vi "Getter.vi"(8 "Error In":errorcluster, 11 "Waypoint In":refnum<class "Waypoint.lvclass">) -> (0 "Error Out":errorcluster, 1 "Coords":T1 {"North" format="%#_10f"; "East" format="%#_8f"}, 2 "Tolerance (meters?)":dbl, 3 "Waypoint Out":refnum<class "Waypoint.lvclass">, 5 "Done?":bool)   [LabVIEW 2013, in "Waypoint.lvclass"]
doc: "A getter vi for waypoint class\n\nMac-I Crowell\nJanuray 2014"
uses:
  Waypoint.lvclass
  Data/TypeDefs/UTM Location.ctl
  Waypoint.lvclass/Waypoint.ctl
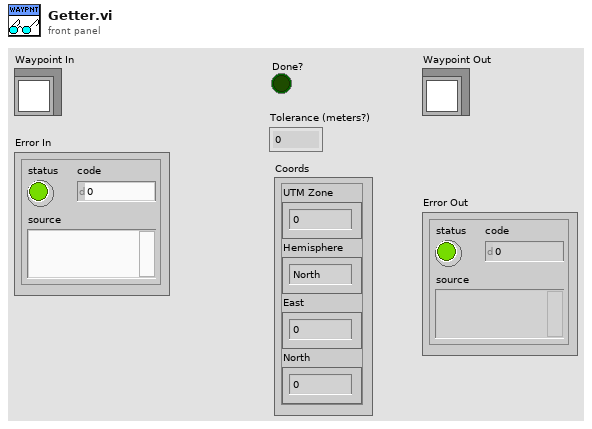
[diagram p1: front panel]
types:
  T1 = typedef "UTM Location.ctl" = cluster{"UTM Zone":dbl, "Hemisphere":enum16{"North", "South"}, "East":dbl, "North":dbl}
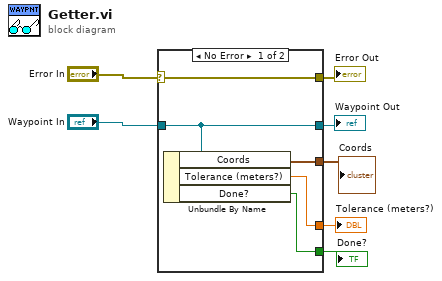
[diagram p0: block diagram]
diagram:
  n1 = case shown="No Error" "Error In" {
    selector: "Error In" -> [w12 w13]
    tunnel: [w12 w13] -> w5
    tunnel: "Waypoint In" -> [w11 w14]
    tunnel: [w11 w14] -> w7
    tunnel: [w10 _] -> w1
    tunnel: [w9 _] -> w3
    tunnel: [w8 _] -> w2
    frame No Error {
      n2 = Unbundle By Name(w11) -> ("Coords"=w10:T1, "Tolerance (meters?)"=w8:dbl, "Done?"=w9:bool)
    }
    frame Error {
    }
  }
  "Waypoint Out" <- w7
  "Error Out" <- w5
  "Done?" <- w3
  "Tolerance (meters?)" <- w2
  "Coords" <- w1
